vi "SRV_Execute Multiple Motor Control Commands.vi"(0 "SRV":refnum<k5>, 1 "Motor Type":T1, 7 "Motor Control Commands":T2[](array[typedef]) {"Value" format="%02x"; "Register" format="%02x"; "I2C Address" format="%02x"}, 11 "error in (no error)":errorcluster) -> (4 "SRV Out":refnum<k5>, 10 "Active Array":bool[](array[boolean]), 15 "error out":errorcluster)   [LabVIEW 2009]
doc: "Author: Mike Schultz (LogicPD, Inc)"
uses:
  Motors Config/SRV_Motor Control Command Config.ctl
  Motors Config/SRV_Motor Legos-Servo.ctl
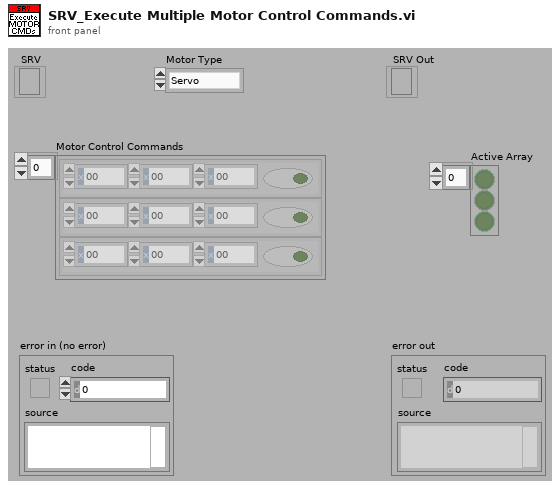
[diagram p1: front panel]
types:
  T1 = typedef "SRV_Motor Legos-Servo.ctl" = enum16{"Servo", "Legos", "Shared Var"}
  T2 = typedef "SRV_Motor Control Command Config.ctl" = cluster{"I2C Address":u8, "Register":u8, "Value":u8, "Active":bool}
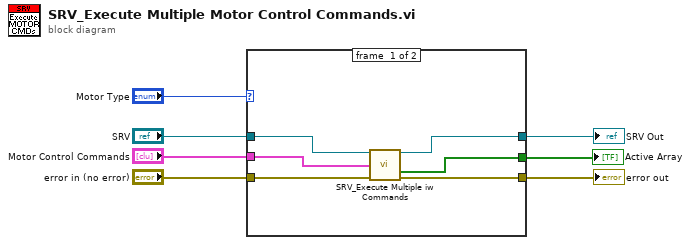
[diagram p0: block diagram]
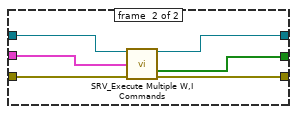
[diagram p2: hidden frame]
diagram:
  n1 = case shown="\"Shared Var\"" "Motor Type" {
    tunnel: "SRV" -> [w13 w16]
    tunnel: [w12 w15] -> w6
    tunnel: [w11 w14] -> w5
    tunnel: [w10 w18] -> w4
    tunnel: "error in (no error)" -> [w9 w19]
    tunnel: "Motor Control Commands" -> [w8 w17]
    frame #0 {
      n2 = call "SRV_Execute Multiple iw Commands.vi"("SRV"=w13, "Motor Control Commands"=w8, "error in (no error)"=w9) -> ("SRV Out"=w12:refnum<k5>, "Active Array"=w11:bool[], "error out"=w10:errorcluster)  [unwired: 10 in]
    }
    frame #1 {
      n3 = call "SRV_Execute Multiple W,I Commands.vi"("SRV"=w16, "Motor Control Commands"=w17, "error in (no error)"=w19) -> ("SRV Out"=w15:refnum<k5>, "Active Array"=w14:bool[], "error out"=w18:errorcluster)  [unwired: 10 in]
    }
  }
  "SRV Out" <- w6
  "error out" <- w4
  "Active Array" <- w5
